vi "ConvertCartesianPosition.vi"(10 "Cartesian position":refnum<k24>, 11 "error in (no error)":errorcluster) -> (2 "Cartesian position":T1, 3 "error out":errorcluster)   [LabVIEW 2019, in "UnderAutomation.Fanuc.lvlib"]
uses:
  UnderAutomation.Fanuc.lvlib
  C:/Users/fg/Documents/Fanuc.vi/LabVIEW_2024/UnderAutomation.Fanuc/lib/UnderAutomation.Fanuc.dll
  LabVIEW_2024/UnderAutomation.Fanuc/lib/UnderAutomation.Fanuc.dll
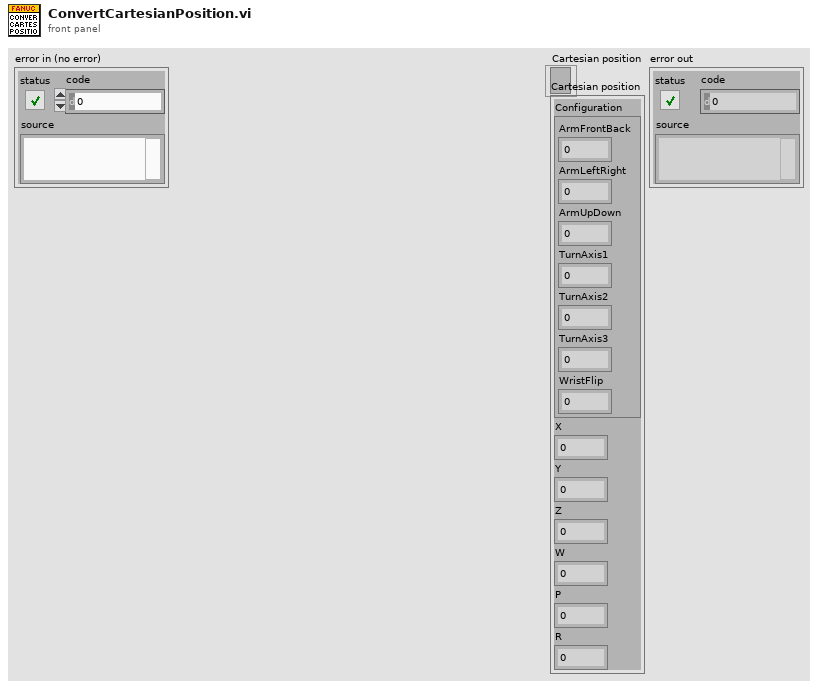
[diagram p1: front panel]
types:
  T1 = cluster{"Configuration":cluster{"ArmFrontBack":i32, "ArmLeftRight":i32, "ArmUpDown":i32, "TurnAxis1":i32, "TurnAxis2":i32, "TurnAxis3":i32, "WristFlip":i32}, "X":dbl, "Y":dbl, "Z":dbl, "W":dbl, "P":dbl, "R":dbl}
  T2 = cluster{"ArmFrontBack":i32, "ArmLeftRight":i32, "ArmUpDown":i32, "TurnAxis1":i32, "TurnAxis2":i32, "TurnAxis3":i32, "WristFlip":i32}
  T3 = cluster{cluster{"ArmFrontBack":i32, "ArmLeftRight":i32, "ArmUpDown":i32, "TurnAxis1":i32, "TurnAxis2":i32, "TurnAxis3":i32, "WristFlip":i32}, "X":dbl, "Y":dbl, "Z":dbl, "W":dbl, "P":dbl, "R":dbl}
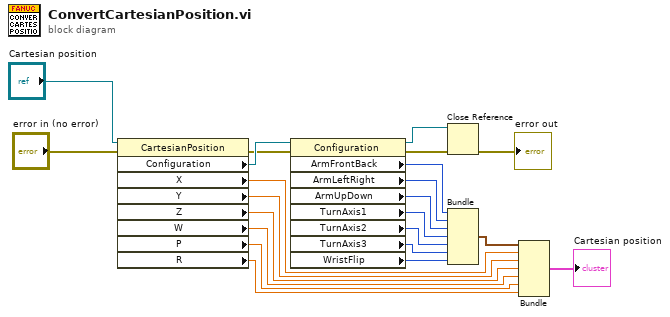
[diagram p0: block diagram]
diagram:
  n1 = property class="CartesianPosition"(reference="Cartesian position", error in="error in (no error)") -> (error out=w4:errorcluster, "Configuration"=w22:refnum<k24>, "X"=w13:dbl, "Y"=w12:dbl, "Z"=w11:dbl, "W"=w10:dbl, "P"=w9:dbl, "R"=w8:dbl)  [unwired: 1 out]
  n2 = property class="Configuration"(reference=w22, error in=w4) -> (reference out=w3:refnum<k24>, error out=w2:errorcluster, "ArmFrontBack"=w21:i32, "ArmLeftRight"=w20:i32, "ArmUpDown"=w19:i32, "TurnAxis1"=w18:i32, "TurnAxis2"=w17:i32, "TurnAxis3"=w16:i32, "WristFlip"=w15:i32)
  n3 = Close Reference(reference=w3, error in (no error)=w2) -> (error out=→"error out":errorcluster)
  n4 = Bundle("ArmFrontBack"=w21, "ArmLeftRight"=w20, "ArmUpDown"=w19, "TurnAxis1"=w18, "TurnAxis2"=w17, "TurnAxis3"=w16, "WristFlip"=w15) -> (w14:T2)  [unwired: 1 in]
  n5 = Bundle(w14, "X"=w13, "Y"=w12, "Z"=w11, "W"=w10, "P"=w9, "R"=w8) -> (→"Cartesian position":T3)  [unwired: 1 in]
